vi "Multicast_Receiver.vi"() -> ()   [LabVIEW 2015]
uses:
  <vilib>/Utility/tcp.llb/UDP Multicast Read-Write Open.vi
panel:
  in  "Tab Control":enum32{"Charts"}(tab)
  out "Translation":dbl[][](graph)
  out "y":dbl
  out "z":dbl
  out "x":dbl
  in  "Stop":bool
  out "roll":dbl
  out "pitch":dbl
  out "yaw":dbl
  out "Rotation":dbl[][](graph)
  out "error out":errorcluster
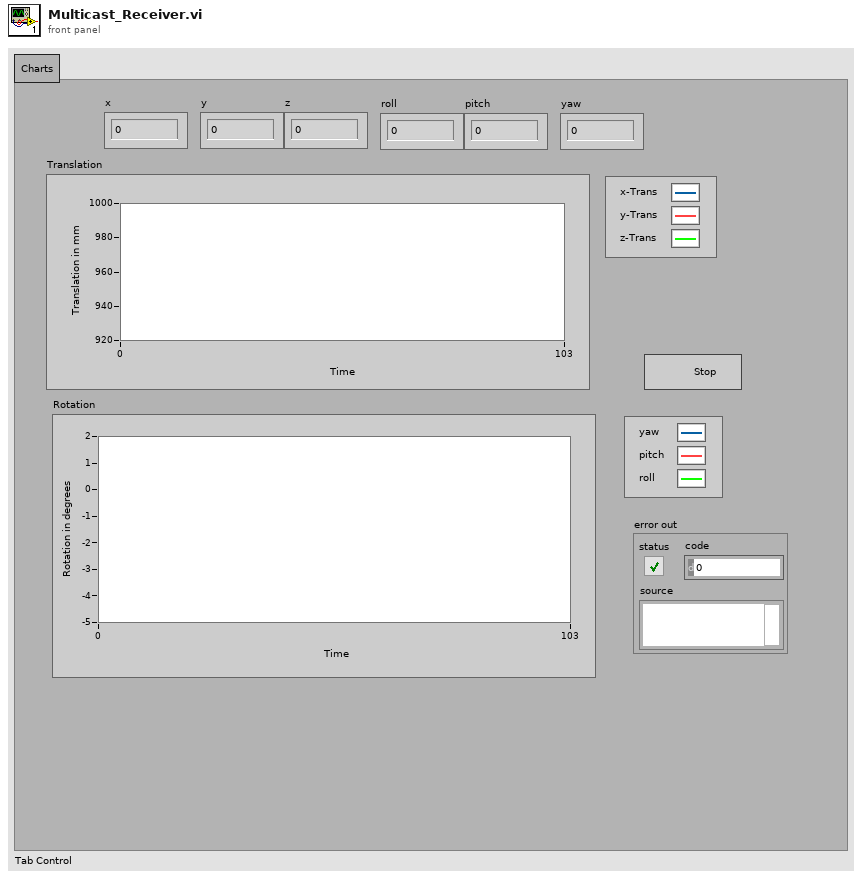
[diagram p1: front panel]
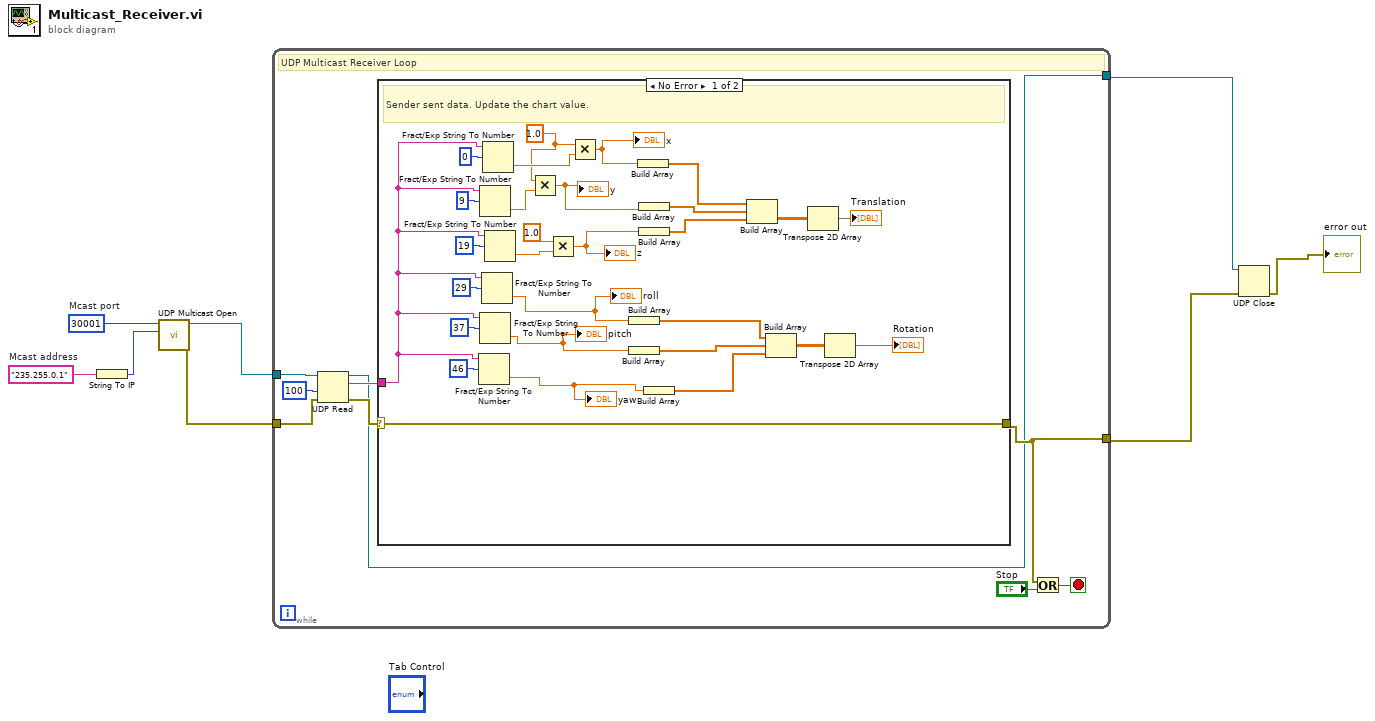
[diagram p0: block diagram]
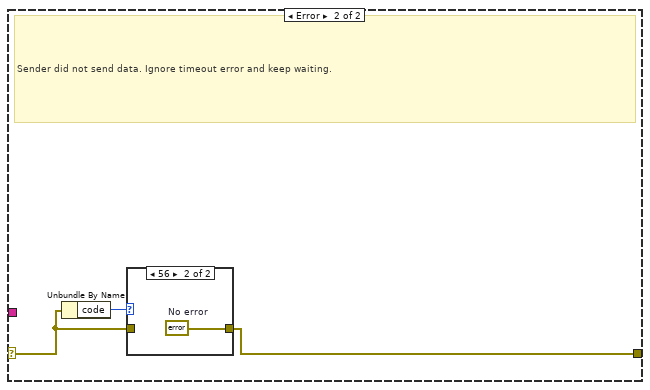
[diagram p2: hidden frame]
diagram:
  w3 = u16 30001  # Mcast port
  w7 = "235.255.0.1"  # Mcast address
  n1 = String To IP(1:w7) -> (0:w2:u32)
  n2 = call-poly <vilib>:"UDP Multicast Open.vi"("multicast addr"=w2, "port"=w3) -> ("error out"=w5:errorcluster, "connection ID"=w4:refnum<k16>)  [unwired: 7 in, 1 out]
  n3 = while {
    tunnel: w4 -> [w17]
    tunnel: [w9] -> w8
    tunnel: w5 -> [w14]
    tunnel: [w10] -> w6
    stop <- w15 stop-if-true
    # "UDP Multicast Receiver Loop"
    n4 = UDP Read(connection ID=w17, timeout ms (25000)=100, 8:w14) -> (data out=w12:string, error out=w11:errorcluster, 3:w9:refnum<k16>)  [unwired: 3 out]
    n5 = case shown="No Error" w11 {
      selector: w11 -> [w46 w48]
      tunnel: w12 -> [w29 _]
      tunnel: [w46 w47] -> w10
      frame No Error {
        w26 = 1.0 ("y")
        # "Sender sent data. Update the chart value."
        n6 = Fract/Exp String To Number(string=w29, offset=46) -> (number=w18:dbl)  [unwired: 2 in, 1 out]
        "yaw" <- w18
        n7 = Fract/Exp String To Number(string=w29, offset=9) -> (number=w23:dbl)  [unwired: 2 in, 1 out]
        n8 = Fract/Exp String To Number(string=w29, offset=37) -> (number=w19:dbl)  [unwired: 2 in, 1 out]
        "pitch" <- w19
        n9 = Fract/Exp String To Number(string=w29, offset=29) -> (number=w20:dbl)  [unwired: 2 in, 1 out]
        "roll" <- w20
        n10 = Fract/Exp String To Number(string=w29, offset=0) -> (number=w27:dbl)  [unwired: 2 in, 1 out]
        n11 = Fract/Exp String To Number(string=w29, offset=19) -> (number=w25:dbl)  [unwired: 2 in, 1 out]
        n12 = Multiply(x=w26, y=w23) -> (x*y=w22:dbl)
        "y" <- w22
        n13 = Multiply(x=1.0, y=w25) -> (x*y=w21:dbl)
        "z" <- w21
        n14 = Multiply(x=w26, y=w27) -> (x*y=w28:dbl)
        "x" <- w28
        n15 = Build Array(w20) -> (w32:dbl[])
        n16 = Build Array(w19) -> (w33:dbl[])
        n17 = Build Array(w28) -> (w36:dbl[])
        n18 = Build Array(w22) -> (w35:dbl[])
        n19 = Build Array(w21) -> (w40:dbl[])
        n20 = Build Array(w18) -> (w34:dbl[])
        n21 = Build Array(w36, w35, w40) -> (w42:dbl[][])
        n22 = Build Array(w32, w33, w34) -> (w31:dbl[][])
        n23 = Transpose 2D Array(2D array=w42) -> (transposed array=→"Translation":dbl[][])
        n24 = Transpose 2D Array(2D array=w31) -> (transposed array=→"Rotation":dbl[][])
      }
      frame Error {
        # "Sender did not send data. Ignore timeout error and keep waiting."
        n25 = Unbundle By Name(w48) -> ("code"=w49:i32)
        n26 = case shown="56" w49 {
          tunnel: w48 -> [w50 _]
          tunnel: [w50 w51] -> w47
          frame Default {
          }
          frame 56 {
            w51 = errorcluster {"status"=FALSE, "code"=0, "source"=""}  # No error
          }
        }
      }
    }
    n27 = Or(x=w10, y="Stop") -> (x .or. y?=w15:bool)
  }
  n28 = UDP Close(connection ID=w8, 8:w6) -> (error out=→"error out":errorcluster)  [unwired: 1 out]
